vi "GPIB Receive.vi"(7 "size":i32, 9 "text":string, 10 "address":i16, 11 "id":i32) -> (1 "text out":string, 3 "function return":u32)   [LabVIEW 2018, in "Copy of Andor SDK.lvlib"]
doc: "EXPNETTYPE unsigned int WINAPI GPIBReceive(int id, short address, char * text, int size);"
uses:
  Copy of Andor SDK.lvlib
  <userlib>/Andor SDK/ATMCD32D.dll
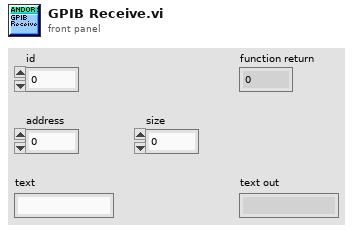
[diagram p1: front panel]
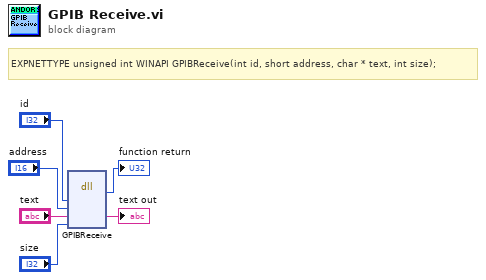
[diagram p0: block diagram]
diagram:
  # "EXPNETTYPE unsigned int WINAPI GPIBReceive(int id, short address, char * text, int size);"
  n1 = dll-call lib="C:/Program Files (x86)/National Instruments/LabVIEW 2018/user.lib/Andor SDK/ATMCD32D.*" fn="GPIBReceive"("id"="id", "address"="address", "text"="text", "size"="size") -> (→"function return":u32, "text"=→"text out":string)  [unwired: 6 in, 2 out]
